vi "数字滤波.vi"() -> ()   [LabVIEW 2019]
uses:
  <vilib>/Analysis/3filter.llb/Butterworth Filter (DBL).vi
  <vilib>/Analysis/NI_AALBase.lvlib
panel:
  in  "停止":bool=TRUE
  out "滤波后的信号":cluster{i32, dbl, dbl[]}(graph)
  out "滤波前的信号":cluster{i32, dbl, dbl[]}(graph)
  in  "阶数":dbl(slide) scale=0.0..10.0
  in  "截止频率":dbl(slide) scale=0.0..50.0
  in  "采样频率":dbl format="%#_13g"
  in  "正弦信号频率":dbl format="%#_13g"
  in  "采样点数":dbl format="%#_13g"
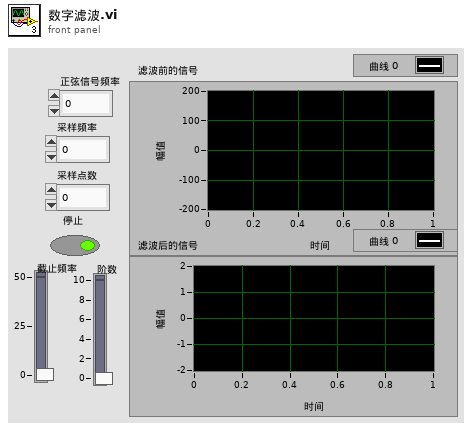
[diagram p1: front panel]
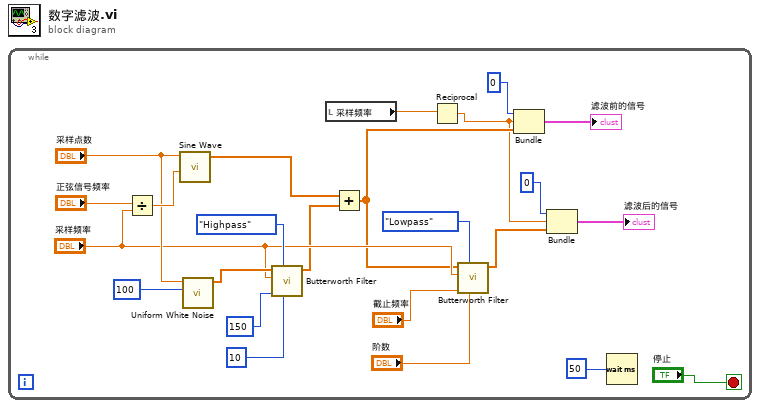
[diagram p0: block diagram]
diagram:
  n1 = while {
    stop <- "停止" stop-if-true
    n2 = Divide(x="正弦信号频率", y="采样频率") -> (x/y=w13:dbl)
    n3 = call <vilib>:"Sine Wave.vi"("samples"="采样点数", "frequency"=w13) -> ("sine wave"=w11:dbl[])  [unwired: 3 in, 2 out]
    n4 = call <vilib>:"Uniform White Noise.vi"("amplitude"=100, "samples"="采样点数") -> ("uniform white noise"=w10:dbl[])  [unwired: 8 in, 1 out]
    n5 = call-poly <vilib>:"Butterworth Filter.vi"("order"=10, "filter type"=enum16{"Lowpass", "Highpass"}."Highpass", "low cutoff freq: fl"=150, "sampling freq: fs"="采样频率", "X"=w10) -> ("Filtered X"=w8:dbl[])  [unwired: 3 in, 1 out]
    n6 = local read "采样频率"() -> (w15:dbl)
    n7 = Add(x=w11, y=w8) -> (x+y=w7:dbl[])
    n8 = Reciprocal(x=w15) -> (1/x=w6:dbl)
    n9 = call-poly <vilib>:"Butterworth Filter.vi"("order"="阶数", "filter type"=enum16{"Lowpass", "Highpass"}."Lowpass", "low cutoff freq: fl"="截止频率", "sampling freq: fs"="采样频率", "X"=w7) -> ("Filtered X"=w5:dbl[])  [unwired: 3 in, 1 out]
    n10 = Bundle(0, w6, w7) -> (→"滤波前的信号":cluster{i32, dbl, dbl[]})  [unwired: 1 in]
    n11 = Bundle(0, w6, "Filtered X"=w5) -> (→"滤波后的信号":cluster{i32, dbl, "Filtered X":dbl[]})  [unwired: 1 in]
    n12 = Wait (ms)(milliseconds to wait=50) -> ()  [unwired: 1 out]
  }
